vi "Set Pump State.vi"(8 "error in (no error)":errorcluster, 10 "Pump State":bool, 11 "HW Evaporative Cooler in":refnum<class "HW Evaporative Cooler.lvclass">) -> (0 "error out":errorcluster)   [LabVIEW 2018, in "HW Evaporative Cooler.lvclass"]
uses:
  HW Evaporative Cooler.lvclass
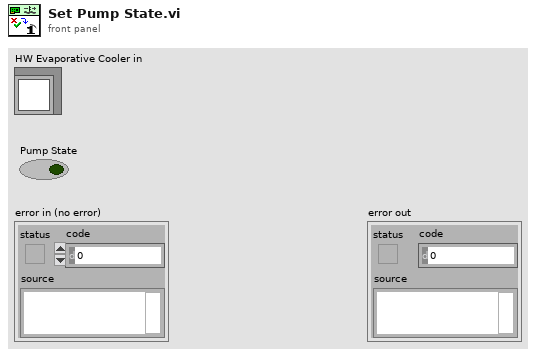
[diagram p1: front panel]
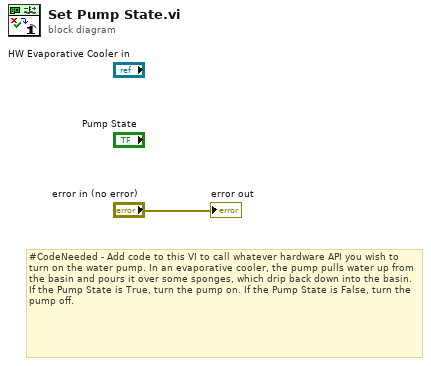
[diagram p0: block diagram]
diagram:
  # "#CodeNeeded - Add code to this VI to call whatever hardware API you wish to turn on the water pump. In an evaporative cooler, the pump pulls water up from the basin and pours it over some sponges, which drip back down into the basin. If the Pump State is True, turn the pump on. If the Pump State is False, turn the pump off."
  "error out" <- "error in (no error)"
